vi "ad discrete outv.vi"(0 "adh":i32, 1 "datav":u64[](array[numeric])=array[4097 elements], 5 "chac":i32, 7 "chav":i32[](array[numeric])=array[4097 elements], 9 "rangev":u64[](array[numeric])=array[4097 elements], 11 "error in (no error)":errorcluster) -> (4 "function return":i32, 15 "error out":errorcluster)   [LabVIEW 2021, in "libad4.lvlib"]
doc: "LIBAD4 function: ad_discrete_outv (int32_t adh, int32_t chac, int32_t chav[], uint64_t rangev[], uint64_t datav[]);\n\nThe ad_discrete_outv() function sets chac outputs at once no matter if analog or digital."
uses:
  <userlib>/libad4/libad4.lvlib
  <userlib>/libad4/libad4.dll
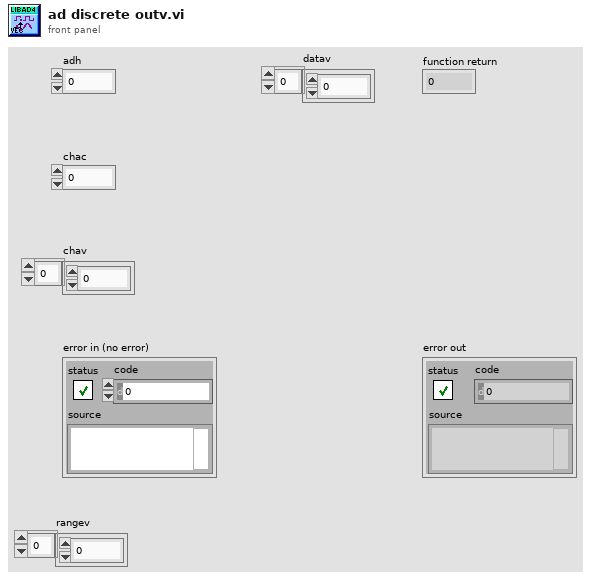
[diagram p1: front panel]
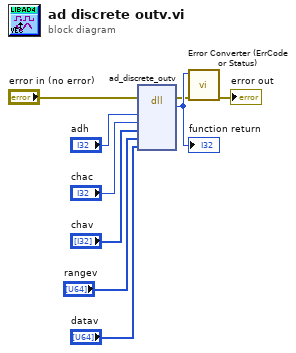
[diagram p0: block diagram]
diagram:
  n1 = dll-call lib="C:/Program Files/National Instruments/LabVIEW 2021/user.lib/libad4/libad4.*" fn="ad_discrete_outv"(error in="error in (no error)", "adh"="adh", "chac"="chac", "chav"="chav", "rangev"="rangev", "datav"="datav") -> (error out=w4:errorcluster, "return type"=w9:i32)  [unwired: 7 in, 1 out]
  "function return" <- w9
  n2 = call <userlib>:"Error Converter (ErrCode or Status).vi"("error in (no error)"=w4, "error code"=w9) -> ("error out"=→"error out":errorcluster)  [unwired: 9 in]
